vi "Day 19 - Not Enough Minerals.vi"() -> ()   [LabVIEW 2020, in "AoC 2022.lvlib"]
uses:
  AoC 2022.lvlib
  private/Robot Building Costs.ctl
  private/Cost.ctl
  private/Mineral.ctl
  private/Robot Factory.ctl
  private/Inventory.ctl
  private/Step.ctl
  private/Blueprints.ctl
panel:
  in  "Use This Input":bool
  in  "#Total Time":u32=24
  in  "Time Line":i32(slide) scale=0.0..24.0
  in  "Puzzle Input":string="Blueprint 1: Each ore robot costs 4 ore. Each clay robot costs 2 ore. Each obsidian robot costs 3 ore and 14 clay. Each geode robot costs 2 ore and 7 obsidian.\nBlueprint 2: Each ore robot costs 2 ore. Each clay robot costs 3 ore. Each obsidian robot costs 3 ore and 8 clay. Each geode robot costs 3 ore and 12 obsidian."
  in  "Blueprints":i32(listbox)
  in  "Calculate Steps":bool
  out "Inventory":T1
  out "Robot Factory":T2
  out "Blueprint ID":i32 format="Blueprint %d"
  out "Robot Building Costs":T3 {"Geode"."Mineral" items=["Ore", "Clay", "Obsidian", "Geode", "Open Geode"]; "Obsidian"."Mineral" items=["Ore", "Clay", "Obsidian", "Geode", "Open Geode"]; "Clay"."Mineral" items=["Ore", "Clay", "Obsidian", "Geode", "Open Geode"]; "Ore"."Mineral" items=["Ore", "Clay", "Obsidian", "Geode", "Open Geode"]}
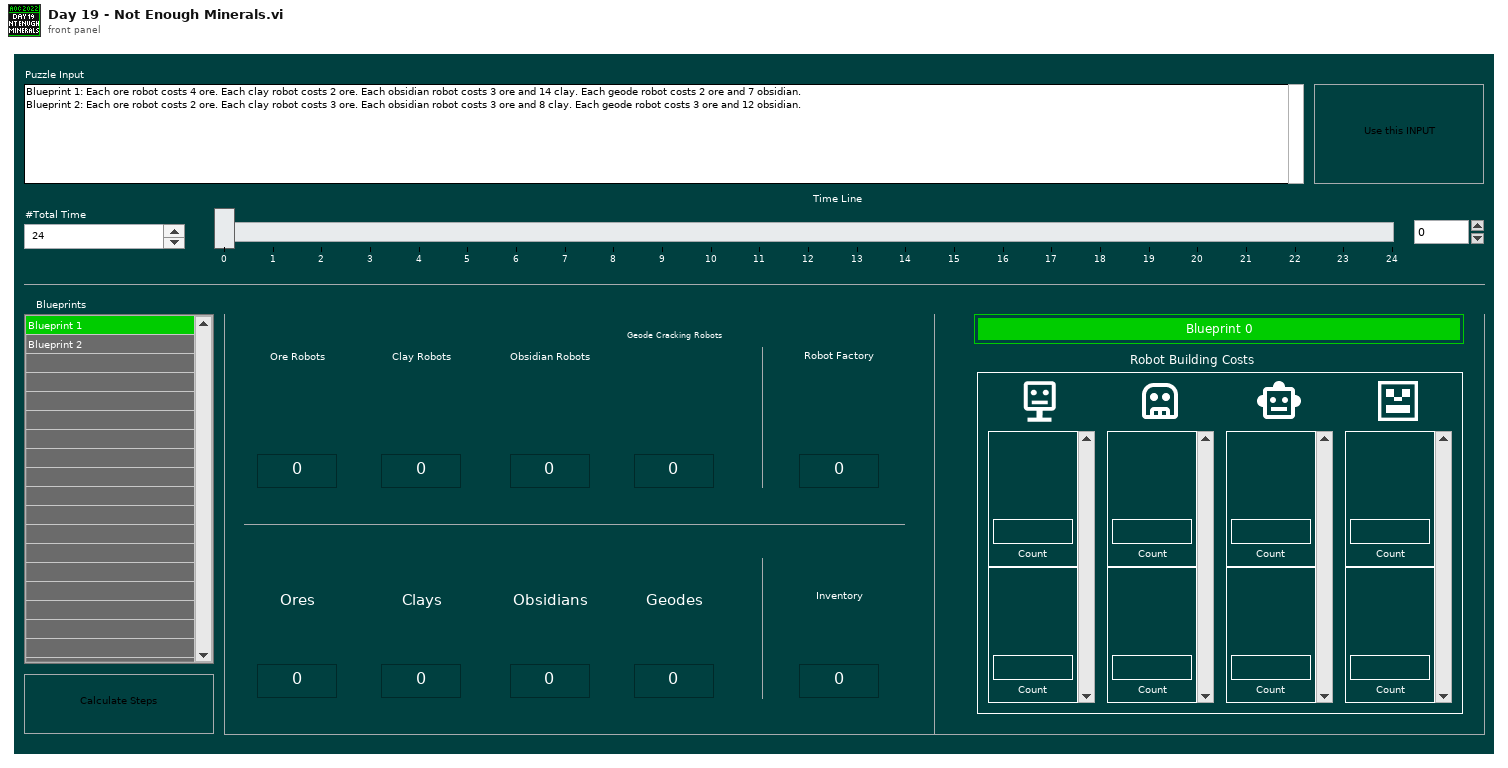
[diagram p1: front panel]
types:
  T1 = typedef "AoC 2022.lvlib/Inventory.ctl" = cluster{"Ores":u32, "Clays":u32, "Obsidians":u32, "Geodes":u32, "Inventory":u32}
  T2 = typedef "AoC 2022.lvlib/Robot Factory.ctl" = cluster{"Ore Robots":u32, "Clay Robots":u32, "Obsidian Robots":u32, "Geode Cracking Robots":u32, "Robot Factory":u32}
  T3 = typedef "AoC 2022.lvlib/Robot Building Costs.ctl" = cluster{"Ore":T4[], "Clay":T4[], "Obsidian":T4[], "Geode":T4[]}
  T4 = typedef "AoC 2022.lvlib/Cost.ctl" = cluster{"Mineral":T5, "Count":u32}
  T5 = typedef "AoC 2022.lvlib/Mineral.ctl" = u16
  T6 = typedef "AoC 2022.lvlib/Blueprints.ctl" = map{i32, T3}
  T7 = typedef "AoC 2022.lvlib/Step.ctl" = cluster{"Inventory":T1, "Robot Factory":T2}
  T8 = cluster{"Puzzle Input":string, "#Total Time":u32, "Time Line":i32, "Blueprints":T6, "Selected Blueprint":i32, "Steps":map{string, T7}}
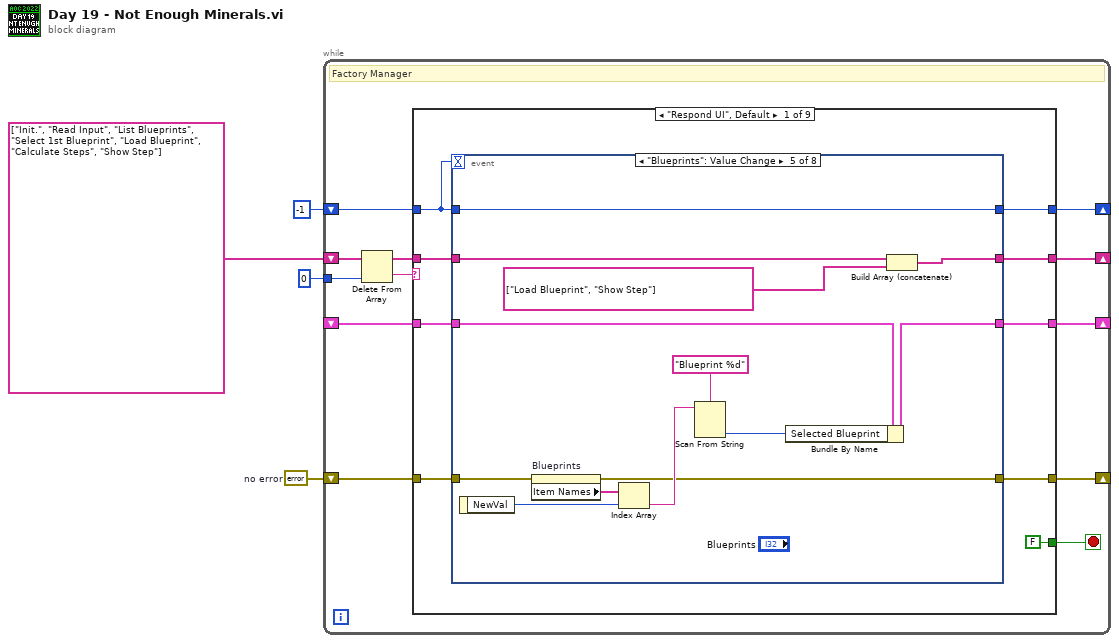
[diagram p0: block diagram]
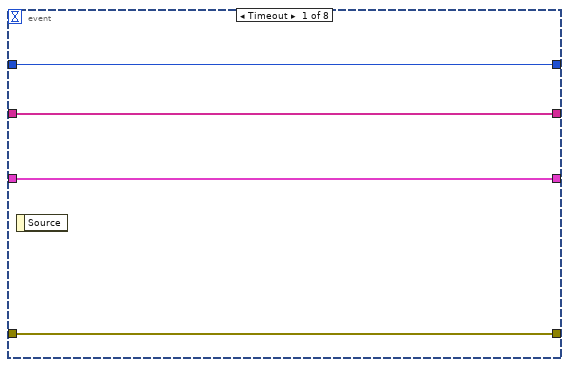
[diagram p2: hidden frame]
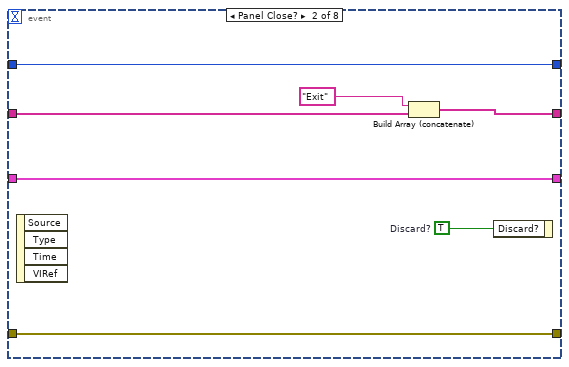
[diagram p3: hidden frame]
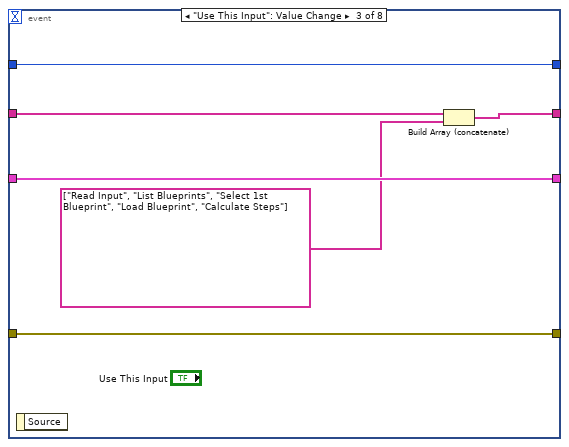
[diagram p4: hidden frame]
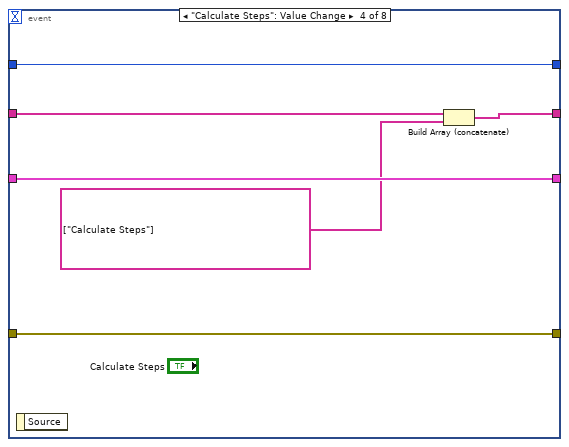
[diagram p5: hidden frame]
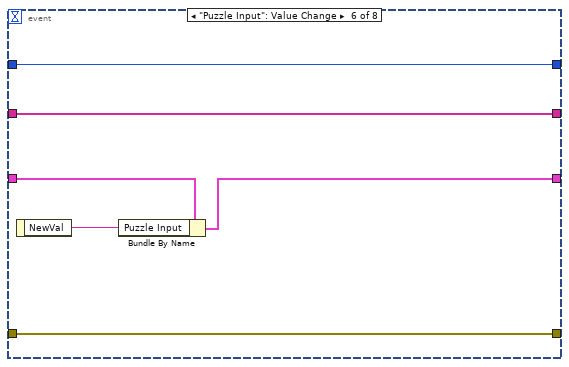
[diagram p6: hidden frame]
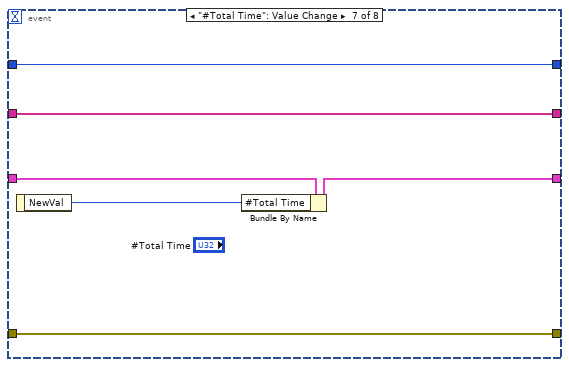
[diagram p7: hidden frame]
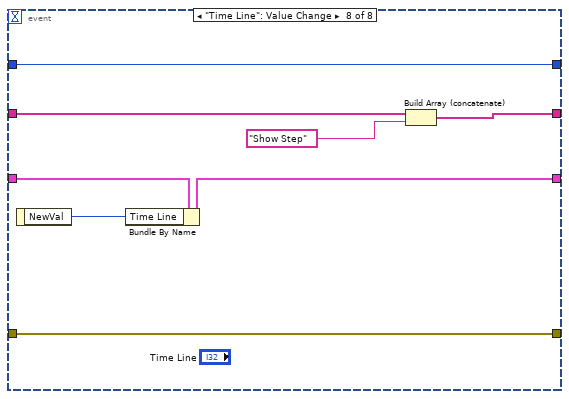
[diagram p8: hidden frame]
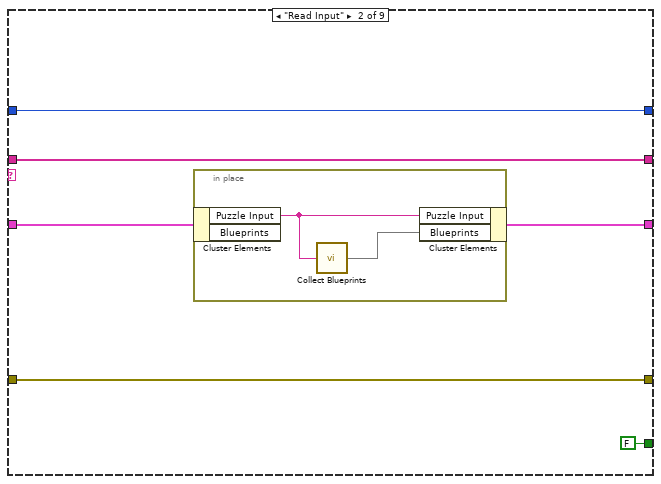
[diagram p9: hidden frame]
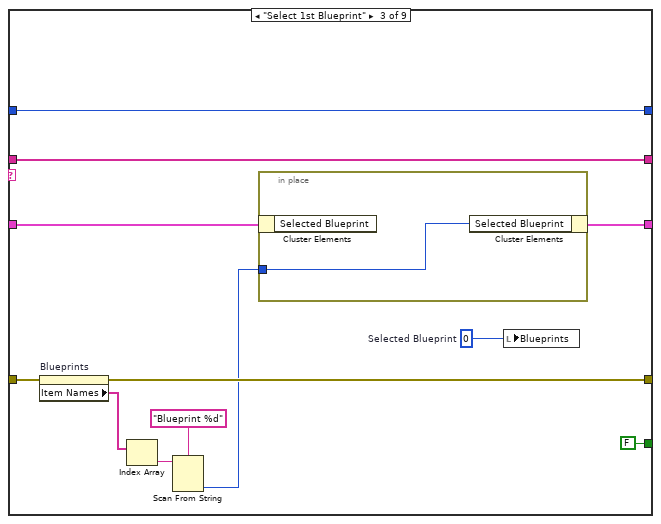
[diagram p10: hidden frame]
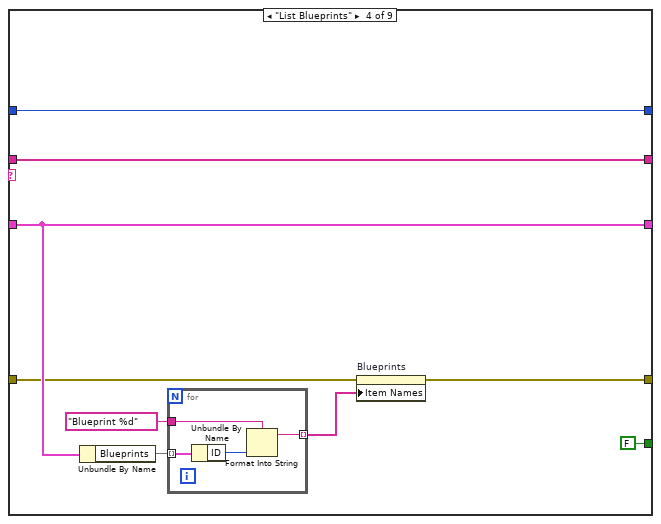
[diagram p11: hidden frame]
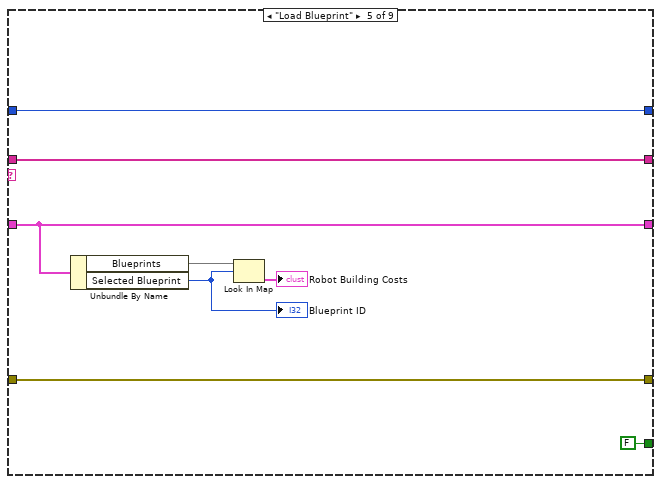
[diagram p12: hidden frame]
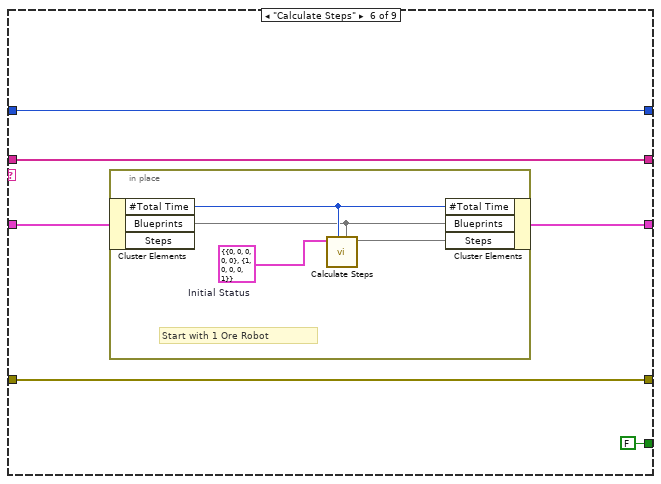
[diagram p13: hidden frame]
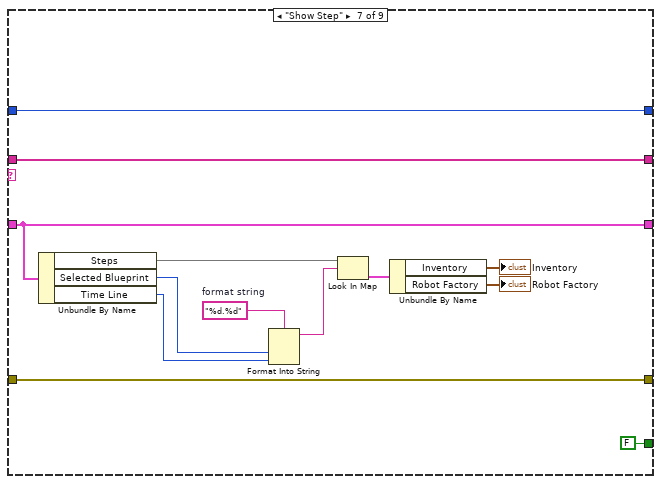
[diagram p14: hidden frame]
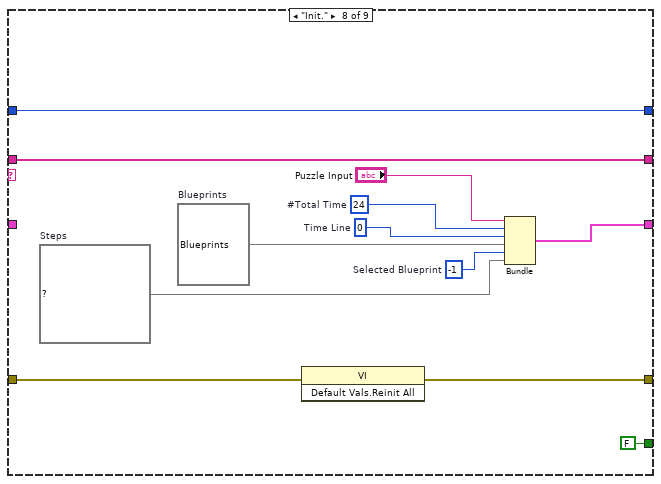
[diagram p15: hidden frame]
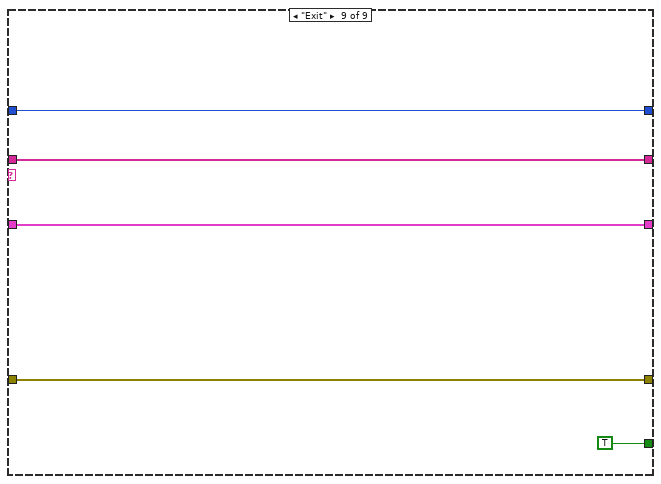
[diagram p16: hidden frame]
diagram:
  w2 = errorcluster {"status"=FALSE, "code"=0, "source"=""}  # no error
  n1 = while {
    shift-right: [w12] -> _
    shift-left: string[] ["Init.", "Read Input", "List Blueprints", "Select 1st Blueprint", "Load Blueprint", "Calculate Steps", "Show Step"] -> [w16]
    shift-right: [w10] -> _
    shift-left: -1 -> [w11]
    shift-right: [w9] -> _
    shift-left: w2 -> [w8]
    tunnel: 0 -> [w7]
    shift-right: [w6] -> _
    shift-left: _ -> [w5]
    stop <- w13 stop-if-true
    # "Factory Manager"
    n2 = Delete From Array(array=w16, index=w7) -> (deleted portion=w15:string, array with subset deleted=w14:string[])  [unwired: 1 in]
    n3 = case shown="\"Respond UI\", Default" w15 {
      tunnel: w14 -> [w21 w87 w101 w111 w123 w129 w146 w158 w162]
      tunnel: [FALSE FALSE FALSE FALSE FALSE FALSE FALSE FALSE TRUE] -> w13
      tunnel: [w22 w87 w101 w111 w123 w129 w146 w158 w162] -> w12
      tunnel: w11 -> [w23 w86 w100 w110 w122 w128 w145 w157 w161]
      tunnel: [w24 w86 w100 w110 w122 w128 w145 w157 w161] -> w10
      tunnel: [w20 w85 w95 w106 w121 w127 w144 w155 w160] -> w9
      tunnel: w8 -> [w19 w85 w96 w107 w121 w127 w144 w154 w160]
      tunnel: [w17 w82 w97 w108 w120 w124 w142 w153 w159] -> w6
      tunnel: w5 -> [w18 w83 w98 w108 w120 w125 w142 _ w159]
      frame "Respond UI", Default {
        n4 = event shown="[4] \"Blueprints\": Value Change" {
          selector: _ -> [_ _ _ _ _ _ _ _]
          dyn-events: _ -> [_ _ _ _ _ _ _ _]
          timeout: w23 -> [_ _ _ _ _ _ _ _]
          tunnel: [w29 w36 w42 w48 w61 w67 w73 w81] -> w24
          tunnel: w23 -> [w29 w36 w42 w48 w61 w67 w73 w81]
          tunnel: [w28 w31 w39 w45 w59 w66 w72 w75] -> w22
          tunnel: w21 -> [w28 w35 w41 w47 w60 w66 w72 w80]
          tunnel: [w27 w34 w40 w46 w53 w65 w71 w79] -> w20
          tunnel: w19 -> [w27 w34 w40 w46 w52 w65 w71 w79]
          tunnel: w18 -> [w26 w33 w38 w44 w58 w64 w70 w78]
          tunnel: [w26 w33 w38 w44 w50 w62 w69 w77] -> w17
          event Timeout {
            n5 = event-data() -> ()  [unwired: 1 in, 1 out]
          }
          event Panel Close? {
            w32 = TRUE  # Discard?
            n6 = event-data() -> ()  [unwired: 1 in, 4 out]
            n7 = Build Array (concatenate)("Exit" ("String"), w35) -> (w31:string[])
            n8 = event-data("Discard?"=w32) -> ()  [unwired: 1 in, 1 out]
          }
          event "Use This Input": Value Change {
            n9 = event-data() -> ()  [unwired: 1 in, 1 out]
            n10 = Build Array (concatenate)(w41, string[] ["Read Input", "List Blueprints", "Select 1st Blueprint", "Load Blueprint", "Calculate Steps"]) -> (w39:string[])
          }
          event "Calculate Steps": Value Change {
            n11 = event-data() -> ()  [unwired: 1 in, 1 out]
            n12 = Build Array (concatenate)(w47, string[] ["Calculate Steps"]) -> (w45:string[])
          }
          event "Blueprints": Value Change {
            n13 = event-data() -> ("NewVal"=w51:i32)  [unwired: 1 in]
            n14 = property on="Blueprints" class="LstBox (strict)"(error in=w52) -> (error out=w53:errorcluster, "Item Names"=w56:string[])  [unwired: 1 in, 1 out]
            n15 = Index Array(array=w56, index=w51) -> (element=w55:string)
            n16 = Scan From String(format string="Blueprint %d", input string=w55) -> (output 1=w49:i32)  [unwired: 3 in, 3 out]
            n17 = Bundle By Name(cluster=w58, "Selected Blueprint"=w49) -> (w50:T8)
            n18 = Build Array (concatenate)(w60, string[] ["Load Blueprint", "Show Step"]) -> (w59:string[])
          }
          event "Puzzle Input": Value Change {
            n19 = event-data() -> ("NewVal"=w63:string)  [unwired: 1 in]
            n20 = Bundle By Name(cluster=w64, "Puzzle Input"=w63) -> (w62:T8)
          }
          event "#Total Time": Value Change {
            n21 = event-data() -> ("NewVal"=w68:u32)  [unwired: 1 in]
            n22 = Bundle By Name(cluster=w70, "#Total Time"=w68) -> (w69:T8)
          }
          event "Time Line": Value Change {
            n23 = event-data() -> ("NewVal"=w76:i32)  [unwired: 1 in]
            n24 = Bundle By Name(cluster=w78, "Time Line"=w76) -> (w77:T8)
            n25 = Build Array (concatenate)(w80, "Show Step" ("String")) -> (w75:string[])
          }
        }
      }
      frame "Read Input" {
        n26 = in-place {
          n27 = in-place-cluster #1(w83) -> ("Puzzle Input"=w88:string)  [unwired: 1 out]
          n28 = call "Collect Blueprints.vi"("Blueprints List"=w88) -> ("Blueprints"=w89:T6)
          n29 = in-place-cluster #1("Puzzle Input"=w88, "Blueprints"=w89) -> (w82:T8)
        }
      }
      frame "Select 1st Blueprint" {
        w93 = 0  # Selected Blueprint
        n30 = property on="Blueprints" class="LstBox (strict)"(error in=w96) -> (error out=w95:errorcluster, "Item Names"=w94:string[])  [unwired: 1 in, 1 out]
        n31 = Index Array(array=w94) -> (element=w92:string)  [unwired: 1 in]
        n32 = Scan From String(format string="Blueprint %d", input string=w92) -> (output 1=w91:i32)  [unwired: 3 in, 3 out]
        n33 = in-place {
          in-place-border: w91 -> [w102]
          n34 = in-place-cluster #2(w98) -> ()  [unwired: 1 out]
          n35 = in-place-cluster #2("Selected Blueprint"=w102) -> (w97:T8)
        }
        n36 = local write "Blueprints"(w93) -> ()
      }
      frame "List Blueprints" {
        n37 = Unbundle By Name(w108) -> ("Blueprints"=w105:T6)
        n38 = for {
          tunnel: w105 -> [w115] mode=indexing
          tunnel: "Blueprint %d" -> [w113]
          tunnel: [w112] -> w103 mode=indexing
          n39 = Unbundle By Name(w115) -> ("ID"=w114:i32)
          n40 = Format Into String(format string=w113, w114) -> (resulting string=w112:string)  [unwired: 2 in, 1 out]
        }
        n41 = property on="Blueprints" class="LstBox (strict)"(error in=w107, "Item Names"=w103) -> (error out=w106:errorcluster)  [unwired: 1 in, 1 out]
      }
      frame "Load Blueprint" {
        n42 = Unbundle By Name(w120) -> ("Blueprints"=w119:T6, "Selected Blueprint"=w116:i32)
        "Blueprint ID" <- w116
        n43 = Look In Map(map=w119, key=w116) -> (value=→"Robot Building Costs":T3)  [unwired: 1 in, 1 out]
      }
      frame "Calculate Steps" {
        n44 = in-place {
          w130 = T7 {"Inventory"={"Ores"=0, "Clays"=0, "Obsidians"=0, "Geodes"=0, "Inventory"=0}, "Robot Factory"={"Ore Robots"=1, "Clay Robots"=0, "Obsidian Robots"=0, "Geode Cracking Robots"=0, "Robot Factory"=1}}  # Initial Status
          # "Start with 1 Ore Robot"
          n45 = in-place-cluster #3(w125) -> ("#Total Time"=w133:u32, "Blueprints"=w132:T6)  [unwired: 1 out]
          n46 = call "Calculate Steps.vi"("Blueprints"=w132, "#Total Time"=w133, "Initial Status"=w130) -> ("Steps"=w131:map{string, T7})  [unwired: 6 in]
          n47 = in-place-cluster #3("#Total Time"=w133, "Blueprints"=w132, "Steps"=w131) -> (w124:T8)
        }
      }
      frame "Show Step" {
        w139 = "%d.%d"  # format string
        n48 = Unbundle By Name(w142) -> ("Steps"=w138:map{string, T7}, "Selected Blueprint"=w141:i32, "Time Line"=w140:i32)
        n49 = Format Into String(format string=w139, w141, w140) -> (resulting string=w137:string)  [unwired: 2 in, 1 out]
        n50 = Look In Map(map=w138, key=w137) -> (value=w136:T7)  [unwired: 1 in, 1 out]
        n51 = Unbundle By Name(w136) -> ("Inventory"=→"Inventory":T1, "Robot Factory"=→"Robot Factory":T2)
      }
      frame "Init." {
        w147 = map{string, T7} {}  # Steps
        w149 = -1  # Selected Blueprint
        w150 = T6 {}  # Blueprints
        w151 = 0  # Time Line
        w152 = u32 24  # #Total Time
        n52 = invoke class="VI" method="Default Vals.Reinit All"(error in=w154) -> (error out=w155:errorcluster)  [unwired: 2 in, 2 out]
        n53 = Bundle("Puzzle Input"="Puzzle Input", "#Total Time"=w152, "Time Line"=w151, "Blueprints"=w150, "Selected Blueprint"=w149, "Steps"=w147) -> (w153:T8)  [unwired: 1 in]
      }
      frame "Exit" {
      }
    }
  }
